vi "SetSystemDefinitionPropertyValue_BinaryString.vi"(8 "error in (no error)":errorcluster, 9 "value":string, 10 "property name":string, 11 "BaseNodeType in":refnum<k24>) -> (0 "error out":errorcluster, 3 "BaseNodeType out":refnum<k24>)   [LabVIEW 2016, in "VeriStandTestUtilities.lvlib"]
uses:
  VeriStandTestUtilities.lvlib
  NationalInstruments.VeriStand.SystemStorage
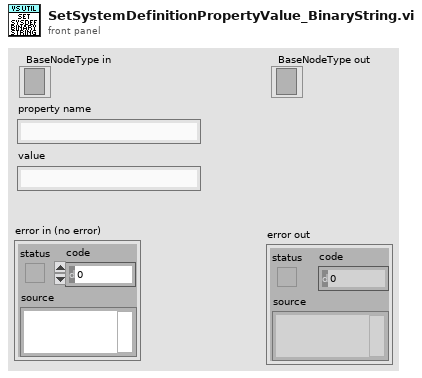
[diagram p1: front panel]
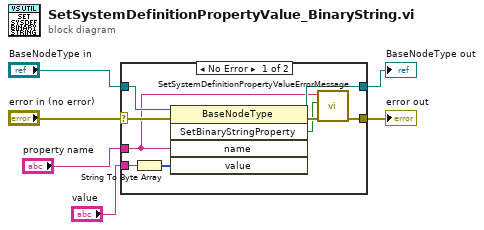
[diagram p0: block diagram]
diagram:
  n1 = case shown="No Error" "error in (no error)" {
    selector: "error in (no error)" -> [w14 w17]
    tunnel: "BaseNodeType in" -> [w15 w16]
    tunnel: "property name" -> [w9 _]
    tunnel: [w13 w16] -> w1
    tunnel: [w11 w17] -> w2
    tunnel: "value" -> [w7 _]
    frame No Error {
      n2 = String To Byte Array(string=w7) -> (unsigned byte array=w8:u8[])
      n3 = invoke class="BaseNodeType" method="SetBinaryStringProperty"(reference=w15, error in=w14, "name"=w9, "value"=w8) -> (reference out=w13:refnum<k24>, error out=w12:errorcluster, "SetBinaryStringProperty"=w10:bool)  [unwired: 1 in, 2 out]
      n4 = call "SetSystemDefinitionPropertyValueErrorMessage.vi"("error in (no error)"=w12, "successful?"=w10, "property name"=w9) -> ("error out"=w11:errorcluster)  [unwired: 8 in]
    }
    frame Error {
    }
  }
  "error out" <- w2
  "BaseNodeType out" <- w1
